vi "Drive_Open6CANMotor.vi"(6 "RightSlaveID2":u8, 7 "LeftSlaveID2":u8, 8 "RightSlaveID1":u8, 9 "RightMasterID":u8, 10 "LeftSlaveID1":u8, 11 "LeftMasterID":u8) -> ()   [LabVIEW 2016]
uses:
  <vilib>/Rock Robotics/WPI/ThirdParty/CanMotor/TalonSRX/WPI_CANTalonSRX_APIControlMode.ctl
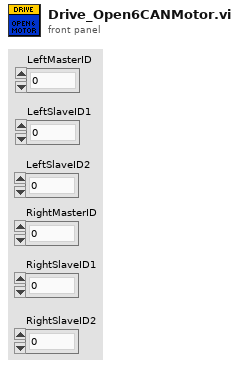
[diagram p1: front panel]
types:
  T1 = typedef "WPI_CANTalonSRX_APIControlMode.ctl" = enum8{"Percent VBus", "Speed", "Position", "Slave", "Unchanged / Invalid", "Voltage Compensation", "Current", "Motion Profile", "Motion Magic"}
  T2 = typedef "WPI_MotorControlDeviceRef.ctl" = cluster{"DeviceStatus":errorcluster, "Type":T3, "PWM":cluster{"PWM Channel":T4, "DeadBand":T5}, "CAN":cluster{"Device Number":u8, "SetOutput VI Ref":variant, "GetOutput VI Ref":variant, "Enable VI Ref":variant, "Disable VI Ref":variant, "Data":variant}, "Invert":bool}
  T3 = typedef "WPI_MotorControlType.ctl" = enum16{"PWM", "CAN"}
  T4 = typedef "FPGA_DIOPWMChannel.ctl" = enum8{"PWM 0", "PWM 1", "PWM 2", "PWM 3", "PWM 4", "PWM 5", "PWM 6", "PWM 7", "PWM 8", "PWM 9", "PWM MXP 0", "PWM MXP 1", "PWM MXP 2", "PWM MXP 3", "PWM MXP 4", "PWM MXP 5", "PWM MXP 6", "PWM MXP 7", "PWM MXP 8", "PWM MXP 9", "Invalid"}
  T5 = typedef "WPI_PWMDeadband.ctl" = cluster{"Name":string, "maxPositivePwm":i32, "minPositivePwm":i32, "centerPwm":i32, "maxNegativePwm":i32, "minNegativePwm":i32, "angularRange":u16}
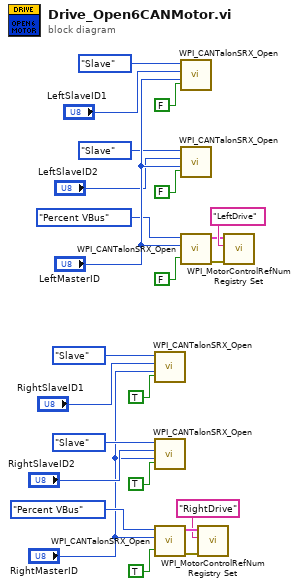
[diagram p0: block diagram]
diagram:
  n1 = call <vilib>:"WPI_CANTalonSRX_Open.vi"("Invert"=TRUE, "Master Device Number"="RightMasterID", "Device Number"="RightSlaveID1", "Control Mode"=WPI_CANTalonSRX_APIControlMode."Slave") -> ()  [unwired: 6 in, 2 out]
  n2 = call <vilib>:"WPI_CANTalonSRX_Open.vi"("Invert"=TRUE, "Master Device Number"="RightMasterID", "Device Number"="RightSlaveID2", "Control Mode"=WPI_CANTalonSRX_APIControlMode."Slave") -> ()  [unwired: 6 in, 2 out]
  n3 = call <vilib>:"WPI_CANTalonSRX_Open.vi"("Invert"=TRUE, "Device Number"="RightMasterID", "Control Mode"=WPI_CANTalonSRX_APIControlMode."Percent VBus") -> ("error out"=w19:errorcluster, "CAN Talon SRX Ref"=w20:T2)  [unwired: 7 in]
  n4 = call <vilib>:"WPI_CANTalonSRX_Open.vi"("Invert"=FALSE, "Master Device Number"="LeftMasterID", "Device Number"="LeftSlaveID1", "Control Mode"=WPI_CANTalonSRX_APIControlMode."Slave") -> ()  [unwired: 6 in, 2 out]
  n5 = call <vilib>:"WPI_CANTalonSRX_Open.vi"("Invert"=FALSE, "Master Device Number"="LeftMasterID", "Device Number"="LeftSlaveID2", "Control Mode"=WPI_CANTalonSRX_APIControlMode."Slave") -> ()  [unwired: 6 in, 2 out]
  n6 = call <vilib>:"WPI_CANTalonSRX_Open.vi"("Invert"=FALSE, "Device Number"="LeftMasterID", "Control Mode"=WPI_CANTalonSRX_APIControlMode."Percent VBus") -> ("error out"=w6:errorcluster, "CAN Talon SRX Ref"=w5:T2)  [unwired: 7 in]
  n7 = call <vilib>:"WPI_MotorControlRefNum Registry Set.vi"("error in (no error)"=w19, "refnum name"="RightDrive", "MotorControlDevRef"=w20) -> ()  [unwired: 7 in, 2 out]
  n8 = call <vilib>:"WPI_MotorControlRefNum Registry Set.vi"("error in (no error)"=w6, "refnum name"="LeftDrive", "MotorControlDevRef"=w5) -> ()  [unwired: 7 in, 2 out]
